vi "Exam.vi"() -> ()   [LabVIEW 2019]
panel:
  out "Timer4":u8
  out "Timer3":u8
  out "Timer2":u8
  out "Timer1":u8
  out "Signal1 4":cluster{"Red":bool, "Amber":bool, "Green":bool}
  out "Signal1 3":cluster{"Red":bool, "Amber":bool, "Green":bool}
  out "Signal1 2":cluster{"Red":bool, "Amber":bool, "Green":bool}
  out "Signal1":cluster{"Red":bool, "Amber":bool, "Green":bool}
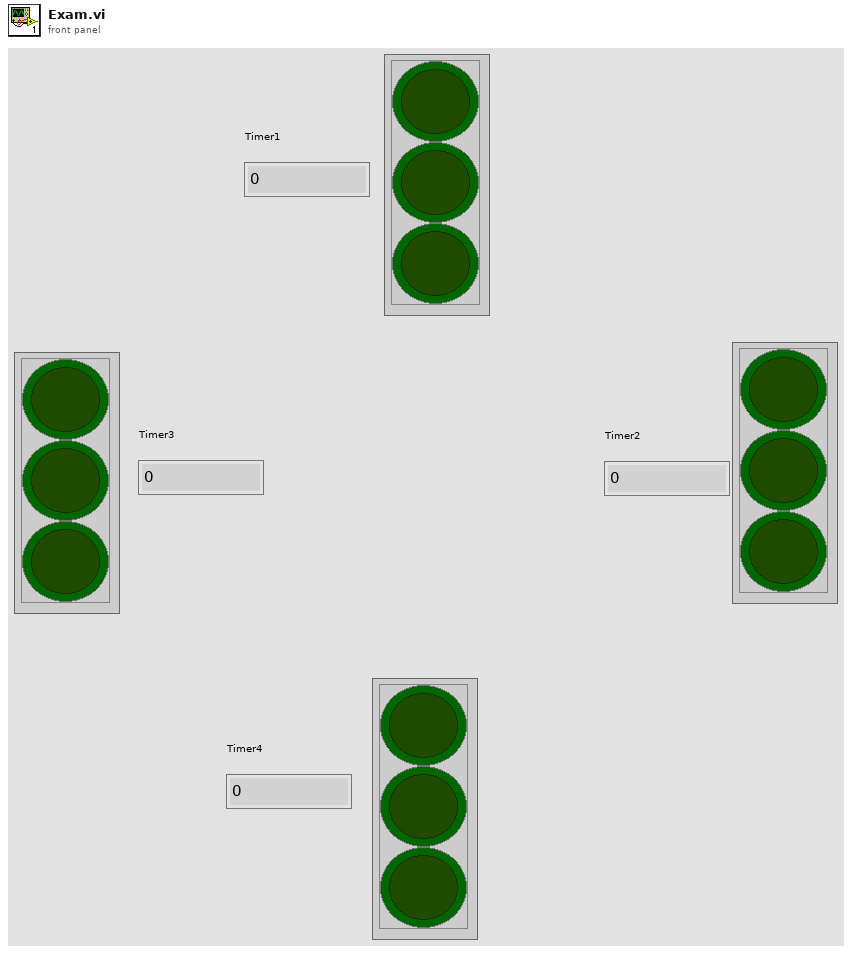
[diagram p1: front panel]
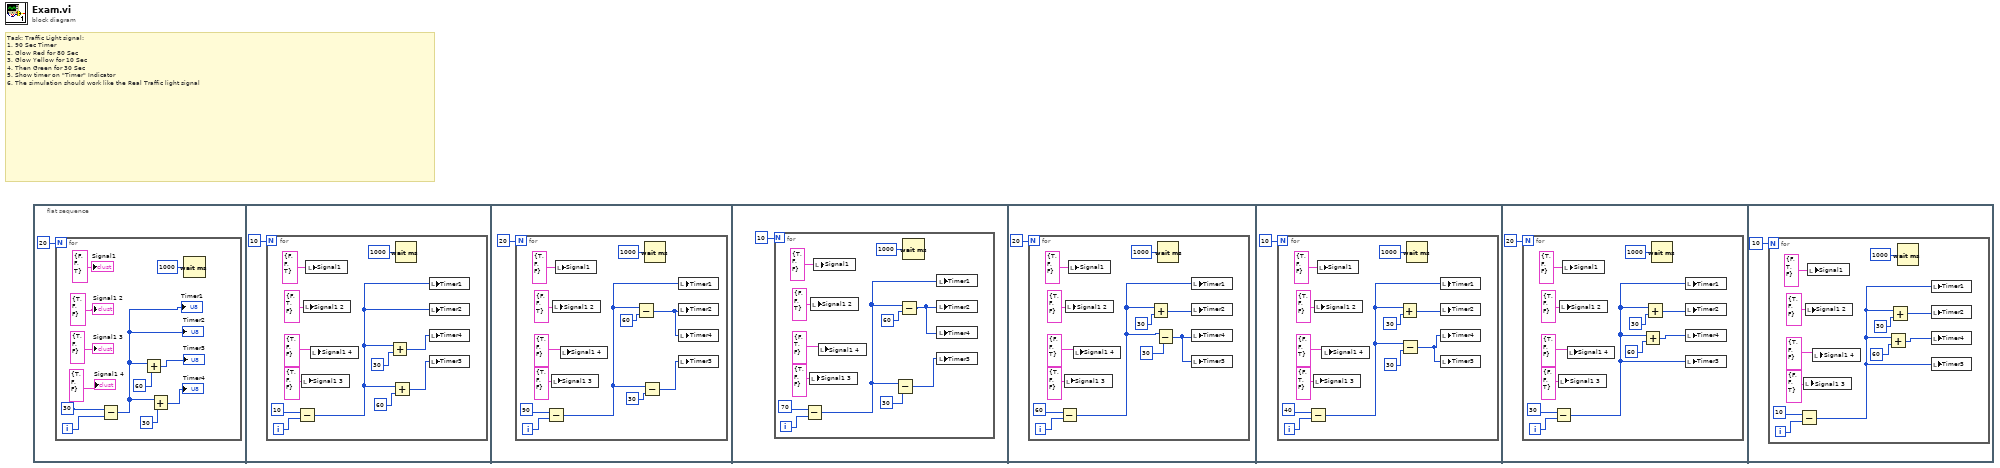
[diagram p0: block diagram]
diagram:
  # "Task: Traffic Light signal:\n1. 90 Sec Timer\n2. Glow Red for 80 Sec\n3. Glow Yellow for 10 Sec\n4. Then Green for 30 Sec\n5. Show timer on \"Timer\" Indicator\n6. The simulation should work like the Real Traffic light signal"
  n1 = flat-sequence {
    frame #0 {
      n2 = for {
        N: 20 -> [_]
        i -> [w8]
        n3 = Subtract(x=30, y=w8) -> (x-y=w3:i32)
        "Timer2" <- w3
        "Timer1" <- w3
        n4 = Add(x=w3, y=60) -> (x+y=→"Timer3":i32)
        n5 = Add(x=w3, y=30) -> (x+y=→"Timer4":i32)
        n6 = Wait (ms)(milliseconds to wait=u32 1000) -> ()  [unwired: 1 out]
        "Signal1" <- cluster{"Red":bool, "Amber":bool, "Green":bool} {"Red"=FALSE, "Amber"=FALSE, "Green"=TRUE} ("Signal1")
        "Signal1 2" <- cluster{"Red":bool, "Amber":bool, "Green":bool} {"Red"=TRUE, "Amber"=FALSE, "Green"=FALSE} ("Signal1 2")
        "Signal1 3" <- cluster{"Red":bool, "Amber":bool, "Green":bool} {"Red"=TRUE, "Amber"=FALSE, "Green"=FALSE} ("Signal1 3")
        "Signal1 4" <- cluster{"Red":bool, "Amber":bool, "Green":bool} {"Red"=TRUE, "Amber"=FALSE, "Green"=FALSE} ("Signal1 4")
      }
    }
    frame #1 {
      n7 = for {
        N: 10 -> [_]
        i -> [w21]
        n8 = Subtract(x=10, y=w21) -> (x-y=w16:i32)
        n9 = local write "Signal1 3"(cluster{"Red":bool, "Amber":bool, "Green":bool} {"Red"=TRUE, "Amber"=FALSE, "Green"=FALSE} ("Signal1")) -> ()
        n10 = local write "Signal1 2"(cluster{"Red":bool, "Amber":bool, "Green":bool} {"Red"=FALSE, "Amber"=TRUE, "Green"=FALSE} ("Signal1 3")) -> ()
        n11 = local write "Signal1"(cluster{"Red":bool, "Amber":bool, "Green":bool} {"Red"=FALSE, "Amber"=FALSE, "Green"=TRUE} ("Signal1 4")) -> ()
        n12 = local write "Signal1 4"(cluster{"Red":bool, "Amber":bool, "Green":bool} {"Red"=TRUE, "Amber"=FALSE, "Green"=FALSE} ("Signal1 2")) -> ()
        n13 = Add(x=w16, y=30) -> (x+y=w18:i32)
        n14 = Add(x=w16, y=60) -> (x+y=w15:i32)
        n15 = Wait (ms)(milliseconds to wait=u32 1000) -> ()  [unwired: 1 out]
        n16 = local write "Timer1"(w16) -> ()
        n17 = local write "Timer2"(w16) -> ()
        n18 = local write "Timer4"(w18) -> ()
        n19 = local write "Timer3"(w15) -> ()
      }
    }
    frame #2 {
      n20 = for {
        N: 20 -> [_]
        i -> [w34]
        n21 = Subtract(x=90, y=w34) -> (x-y=w28:i32)
        n22 = local write "Signal1 3"(cluster{"Red":bool, "Amber":bool, "Green":bool} {"Red"=TRUE, "Amber"=FALSE, "Green"=FALSE} ("Signal1")) -> ()
        n23 = local write "Signal1 2"(cluster{"Red":bool, "Amber":bool, "Green":bool} {"Red"=FALSE, "Amber"=FALSE, "Green"=TRUE} ("Signal1 3")) -> ()
        n24 = local write "Signal1"(cluster{"Red":bool, "Amber":bool, "Green":bool} {"Red"=TRUE, "Amber"=FALSE, "Green"=FALSE} ("Signal1 4")) -> ()
        n25 = local write "Signal1 4"(cluster{"Red":bool, "Amber":bool, "Green":bool} {"Red"=TRUE, "Amber"=FALSE, "Green"=FALSE} ("Signal1 2")) -> ()
        n26 = Subtract(x=w28, y=60) -> (x-y=w31:i32)
        n27 = Subtract(x=w28, y=30) -> (x-y=w29:i32)
        n28 = Wait (ms)(milliseconds to wait=u32 1000) -> ()  [unwired: 1 out]
        n29 = local write "Timer1"(w28) -> ()
        n30 = local write "Timer2"(w31) -> ()
        n31 = local write "Timer4"(w31) -> ()
        n32 = local write "Timer3"(w29) -> ()
      }
    }
    frame #3 {
      n33 = for {
        N: 10 -> [_]
        i -> [w47]
        n34 = Subtract(x=70, y=w47) -> (x-y=w42:i32)
        n35 = local write "Signal1 3"(cluster{"Red":bool, "Amber":bool, "Green":bool} {"Red"=TRUE, "Amber"=FALSE, "Green"=FALSE} ("Signal1")) -> ()
        n36 = local write "Signal1 2"(cluster{"Red":bool, "Amber":bool, "Green":bool} {"Red"=FALSE, "Amber"=FALSE, "Green"=TRUE} ("Signal1 3")) -> ()
        n37 = local write "Signal1"(cluster{"Red":bool, "Amber":bool, "Green":bool} {"Red"=TRUE, "Amber"=FALSE, "Green"=FALSE} ("Signal1 4")) -> ()
        n38 = local write "Signal1 4"(cluster{"Red":bool, "Amber":bool, "Green":bool} {"Red"=FALSE, "Amber"=TRUE, "Green"=FALSE} ("Signal1 2")) -> ()
        n39 = Subtract(x=w42, y=30) -> (x-y=w43:i32)
        n40 = Subtract(x=w42, y=60) -> (x-y=w41:i32)
        n41 = Wait (ms)(milliseconds to wait=u32 1000) -> ()  [unwired: 1 out]
        n42 = local write "Timer1"(w42) -> ()
        n43 = local write "Timer2"(w41) -> ()
        n44 = local write "Timer4"(w41) -> ()
        n45 = local write "Timer3"(w43) -> ()
      }
    }
    frame #4 {
      n46 = for {
        N: 20 -> [_]
        i -> [w60]
        n47 = Subtract(x=60, y=w60) -> (x-y=w55:i32)
        n48 = local write "Signal1 3"(cluster{"Red":bool, "Amber":bool, "Green":bool} {"Red"=TRUE, "Amber"=FALSE, "Green"=FALSE} ("Signal1")) -> ()
        n49 = local write "Signal1 2"(cluster{"Red":bool, "Amber":bool, "Green":bool} {"Red"=TRUE, "Amber"=FALSE, "Green"=FALSE} ("Signal1 3")) -> ()
        n50 = local write "Signal1"(cluster{"Red":bool, "Amber":bool, "Green":bool} {"Red"=TRUE, "Amber"=FALSE, "Green"=FALSE} ("Signal1 4")) -> ()
        n51 = local write "Signal1 4"(cluster{"Red":bool, "Amber":bool, "Green":bool} {"Red"=FALSE, "Amber"=FALSE, "Green"=TRUE} ("Signal1 2")) -> ()
        n52 = Add(x=w55, y=30) -> (x+y=w56:i32)
        n53 = Subtract(x=w55, y=30) -> (x-y=w54:i32)
        n54 = Wait (ms)(milliseconds to wait=u32 1000) -> ()  [unwired: 1 out]
        n55 = local write "Timer1"(w55) -> ()
        n56 = local write "Timer2"(w56) -> ()
        n57 = local write "Timer4"(w54) -> ()
        n58 = local write "Timer3"(w54) -> ()
      }
    }
    frame #5 {
      n59 = for {
        N: 10 -> [_]
        i -> [w73]
        n60 = Subtract(x=40, y=w73) -> (x-y=w69:i32)
        n61 = local write "Signal1 3"(cluster{"Red":bool, "Amber":bool, "Green":bool} {"Red"=FALSE, "Amber"=TRUE, "Green"=FALSE} ("Signal1")) -> ()
        n62 = local write "Signal1 2"(cluster{"Red":bool, "Amber":bool, "Green":bool} {"Red"=TRUE, "Amber"=FALSE, "Green"=FALSE} ("Signal1 3")) -> ()
        n63 = local write "Signal1"(cluster{"Red":bool, "Amber":bool, "Green":bool} {"Red"=TRUE, "Amber"=FALSE, "Green"=FALSE} ("Signal1 4")) -> ()
        n64 = local write "Signal1 4"(cluster{"Red":bool, "Amber":bool, "Green":bool} {"Red"=FALSE, "Amber"=FALSE, "Green"=TRUE} ("Signal1 2")) -> ()
        n65 = Add(x=w69, y=30) -> (x+y=w70:i32)
        n66 = Subtract(x=w69, y=30) -> (x-y=w67:i32)
        n67 = Wait (ms)(milliseconds to wait=u32 1000) -> ()  [unwired: 1 out]
        n68 = local write "Timer1"(w69) -> ()
        n69 = local write "Timer2"(w70) -> ()
        n70 = local write "Timer4"(w67) -> ()
        n71 = local write "Timer3"(w67) -> ()
      }
    }
    frame #6 {
      n72 = for {
        N: 20 -> [_]
        i -> [w86]
        n73 = Subtract(x=30, y=w86) -> (x-y=w81:i32)
        n74 = local write "Signal1 3"(cluster{"Red":bool, "Amber":bool, "Green":bool} {"Red"=FALSE, "Amber"=FALSE, "Green"=TRUE} ("Signal1")) -> ()
        n75 = local write "Signal1 2"(cluster{"Red":bool, "Amber":bool, "Green":bool} {"Red"=TRUE, "Amber"=FALSE, "Green"=FALSE} ("Signal1 3")) -> ()
        n76 = local write "Signal1"(cluster{"Red":bool, "Amber":bool, "Green":bool} {"Red"=TRUE, "Amber"=FALSE, "Green"=FALSE} ("Signal1 4")) -> ()
        n77 = local write "Signal1 4"(cluster{"Red":bool, "Amber":bool, "Green":bool} {"Red"=TRUE, "Amber"=FALSE, "Green"=FALSE} ("Signal1 2")) -> ()
        n78 = Add(x=w81, y=60) -> (x+y=w82:i32)
        n79 = Add(x=w81, y=30) -> (x+y=w83:i32)
        n80 = Wait (ms)(milliseconds to wait=u32 1000) -> ()  [unwired: 1 out]
        n81 = local write "Timer1"(w81) -> ()
        n82 = local write "Timer2"(w83) -> ()
        n83 = local write "Timer4"(w82) -> ()
        n84 = local write "Timer3"(w81) -> ()
      }
    }
    frame #7 {
      n85 = for {
        N: 10 -> [_]
        i -> [w99]
        n86 = Subtract(x=10, y=w99) -> (x-y=w94:i32)
        n87 = local write "Signal1 3"(cluster{"Red":bool, "Amber":bool, "Green":bool} {"Red"=FALSE, "Amber"=FALSE, "Green"=TRUE} ("Signal1")) -> ()
        n88 = local write "Signal1 2"(cluster{"Red":bool, "Amber":bool, "Green":bool} {"Red"=TRUE, "Amber"=FALSE, "Green"=FALSE} ("Signal1 3")) -> ()
        n89 = local write "Signal1"(cluster{"Red":bool, "Amber":bool, "Green":bool} {"Red"=FALSE, "Amber"=TRUE, "Green"=FALSE} ("Signal1 4")) -> ()
        n90 = local write "Signal1 4"(cluster{"Red":bool, "Amber":bool, "Green":bool} {"Red"=TRUE, "Amber"=FALSE, "Green"=FALSE} ("Signal1 2")) -> ()
        n91 = Add(x=w94, y=60) -> (x+y=w95:i32)
        n92 = Add(x=w94, y=30) -> (x+y=w96:i32)
        n93 = Wait (ms)(milliseconds to wait=u32 1000) -> ()  [unwired: 1 out]
        n94 = local write "Timer1"(w94) -> ()
        n95 = local write "Timer2"(w96) -> ()
        n96 = local write "Timer4"(w95) -> ()
        n97 = local write "Timer3"(w94) -> ()
      }
    }
  }
